vi "motor blinking.vi"() -> ()   [LabVIEW 2026]
panel:
  in  "stop":bool
  in  "Boolean 2":bool
  out "Boolean":bool
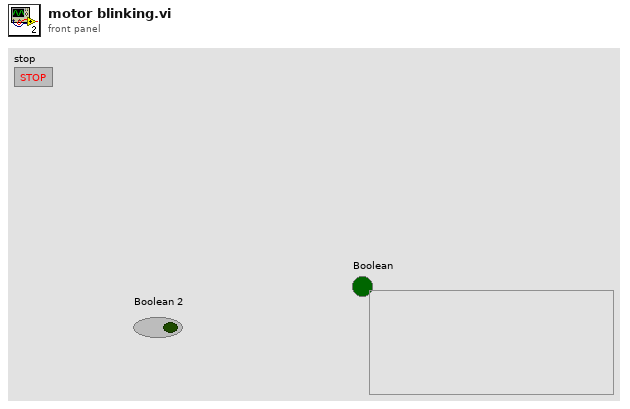
[diagram p1: front panel]
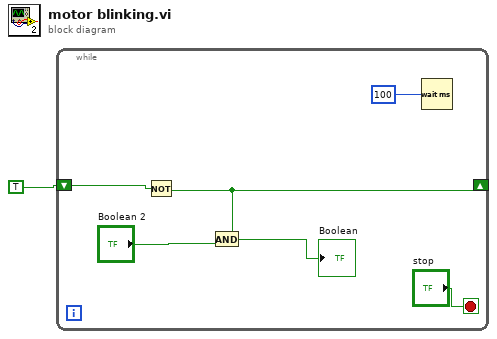
[diagram p0: block diagram]
diagram:
  n1 = while {
    shift-right: [w3] -> _
    shift-left: TRUE -> [w7]
    stop <- "stop" stop-if-true
    n2 = Not(x=w7) -> (.not. x?=w3:bool)
    n3 = And(x=w3, y="Boolean 2") -> (x .and. y?=→"Boolean":bool)
    n4 = Wait (ms)(milliseconds to wait=u32 100) -> ()  [unwired: 1 out]
  }
